vi "write_2d_to_file.vi"(10 "Path 2":path, 11 "Array":u8[][](array[numeric])) -> (3 "refnum out":refnum<file>)   [LabVIEW 2015]
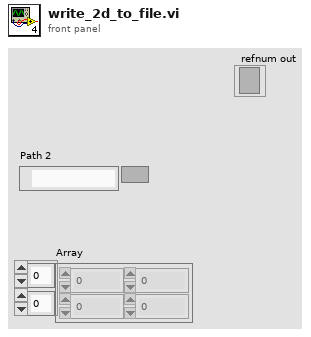
[diagram p1: front panel]
types:
  T1 = enum16{"open", "replace", "create", "open or create", "replace or create", "replace or create with confirmation"}
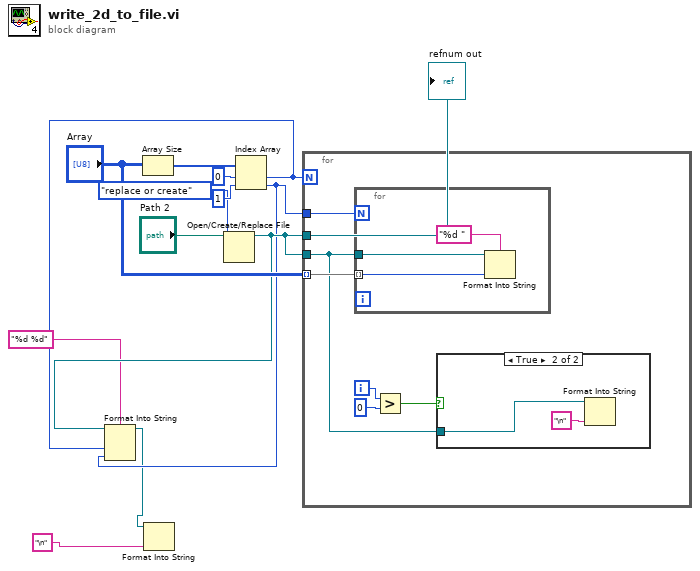
[diagram p0: block diagram]
diagram:
  n1 = Array Size(array="Array") -> (size(s)=w11:i32[])
  n2 = Open/Create/Replace File(file path (use dialog)="Path 2", operation (0:open)=T1."replace or create") -> (refnum out=w6:refnum<file>)  [unwired: 4 in, 2 out]
  "refnum out" <- w6
  n3 = Index Array(array=w11, index #1=0 ("index"), index #2=1 ("index")) -> (element #1=w5:i32, element #2=w3:i32)
  n4 = Format Into String(format string="%d %d", initial string=w6, w5, w3) -> (resulting string=w2:refnum<file>)  [unwired: 1 in, 1 out]
  n5 = Format Into String(initial string=w2, "\n") -> ()  [unwired: 2 in, 2 out]
  n6 = for {
    N: w5 -> [_]
    tunnel: w6 -> [_]
    tunnel: w3 -> [w17]
    tunnel: "Array" -> [w18] mode=indexing
    tunnel: w6 -> [w13]
    i -> [w16]
    n7 = for {
      N: w17 -> [_]
      tunnel: w18 -> [w22] mode=indexing
      tunnel: w13 -> [w21]
      n8 = Format Into String(format string="%d ", initial string=w21, w22) -> ()  [unwired: 1 in, 2 out]
    }
    n9 = Greater?(x=w16, y=0) -> (0:w14:bool)
    n10 = case shown="True" w14 {
      tunnel: w13 -> [_ w19]
      frame False {
      }
      frame True {
        n11 = Format Into String(initial string=w19, "\n") -> ()  [unwired: 2 in, 2 out]
      }
    }
  }
